vi "PH_AxisGUI_6P.PC_Information.vi"(0 "i ref in":refnum<vi>, 1 "quality":i32, 2 "Service Name":string, 3 "Axis Information":T2, 4 "no link":bool, 5 "error in":errorcluster) -> (14 "i ref out":refnum<vi>, 15 "Axis Selector":T1, 16 "Scaled Position":dbl, 19 "error out":errorcluster)   [LabVIEW 2014]
uses:
  PH_AxisGUI_6P.lvlib
  PH_Common/PH_Motion/PH_Motion.Axis State.ctl
  PH_AxisGUI_6P.AxisSelector.ctl
  PH_Common/PH_Motion/PH_Motion.Axis Activity.ctl
  PH_Common/PH_Motion/PH_Motion.Axis Information.ctl
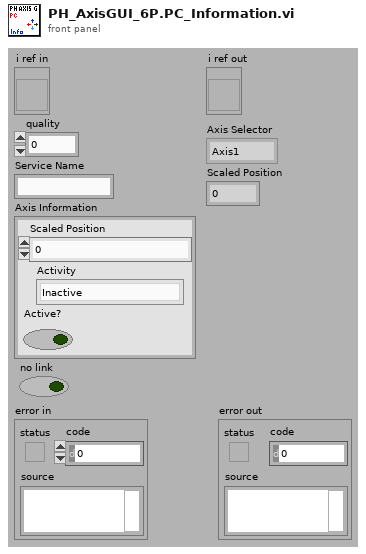
[diagram p1: front panel]
types:
  T1 = typedef "PH_AxisGUI_6P.lvlib/PH_AxisGUI_6P.AxisSelector.ctl" = enum16{"Axis1", "Axis2", "None"}
  T2 = typedef "PH_Motion.Axis Information.ctl" = cluster{"Scaled Position":dbl, "Activity":T3, "Active?":bool}
  T3 = typedef "PH_Motion.Axis Activity.ctl" = enum16{"Inactive", "Ramp", "PI-Controller", "Rotation", "Reference Switch Search", "Reference SwitchSearch", "Mechanical Reference"}
  T4 = typedef "PH_Motion.Axis State.ctl" = enum16{"NoLink", "Inactive", "Active", "Error", "NoInfo"}
  T5 = typedef "PH_AxisGUI_6P.lvlib/PH_AxisGUI_6P.i attribute.ctl" = cluster{"GUI Refs":cluster{"AxisSelection":refnum<vi>, "Tab Control":refnum<vi>}}
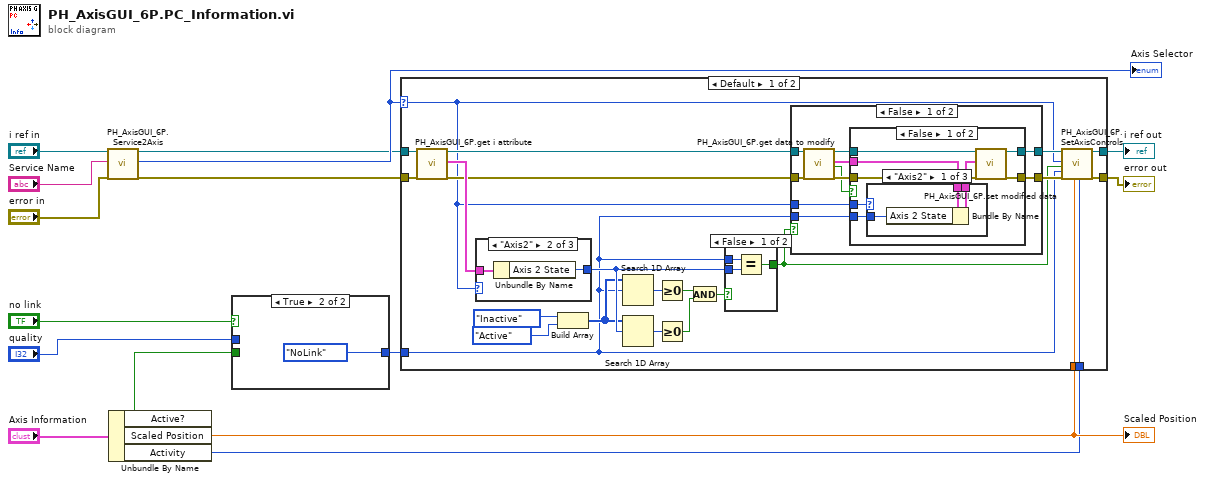
[diagram p0: block diagram]
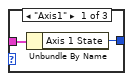
[diagram p2: hidden frame]
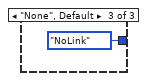
[diagram p3: hidden frame]
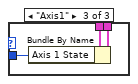
[diagram p5: hidden frame]
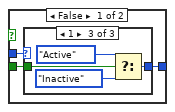
[diagram p10: hidden frame]
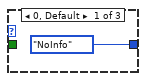
[diagram p11: hidden frame]
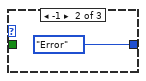
[diagram p12: hidden frame]
diagram:
  n1 = call "PH_AxisGUI_6P.Service2Axis.vi"("i ref in"="i ref in", "service name"="Service Name", "error in"="error in") -> ("i ref out"=w6:refnum<vi>, "Axis Selector"=w7:T1, "error out"=w5:errorcluster)  [unwired: 14 in]
  "Axis Selector" <- w7
  n2 = Unbundle By Name("Axis Information") -> ("Active?"=w10:bool, "Scaled Position"=w4:dbl, "Activity"=w3:T3)
  "Scaled Position" <- w4
  n3 = case "NO LINK?" shown="True" "no link" {
    tunnel: "quality" -> [w17 _]
    tunnel: [w18 PH_Motion.Axis_State."NoLink" ("AxisState")] -> w8
    tunnel: w10 -> [w16 _]
    frame False {
      n4 = case shown="1" w17 {
        tunnel: [PH_Motion.Axis_State."NoInfo" ("AxisState") PH_Motion.Axis_State."Error" ("AxisState") w24] -> w18
        tunnel: w16 -> [_ _ w21]
        frame 0, Default {
        }
        frame -1 {
        }
        frame 1 {
          n5 = Select(t=PH_Motion.Axis_State."Active" ("AxisState"), s=w21, f=PH_Motion.Axis_State."Inactive" ("AxisState")) -> (s? t:f=w24:T4)
        }
      }
    }
    frame True {
    }
  }
  n6 = case shown="Default" w7 {
    selector: w7 -> [w30 _]
    tunnel: w8 -> [w29 _]
    tunnel: w6 -> [w38 w88]
    tunnel: w5 -> [w36 w87]
    tunnel: [w34 w88] -> w1
    tunnel: [w32 w87] -> w2
    tunnel: w4 -> [w27 _]
    tunnel: w3 -> [w26 _]
    frame Default {
      n7 = call "PH_AxisGUI_6P.get i attribute.vi"("i ref in"=w38, "error in (no error)"=w36) -> ("i ref out"=w37:refnum<vi>, "i attribute"=w39:T5, "error out"=w35:errorcluster)  [unwired: 15 in]
      n8 = case shown="\"Axis2\"" w30 {
        tunnel: w39 -> [w50 w52 _]
        tunnel: [w49 w51 PH_Motion.Axis_State."NoLink" ("State")] -> w48
        frame "Axis1" {
          n9 = Unbundle By Name(w50) -> ("Axis 1 State"=w49:T4)
        }
        frame "Axis2" {
          n10 = Unbundle By Name(w52) -> ("Axis 2 State"=w51:T4)
        }
        frame "None", Default {
        }
      }
      n11 = Build Array(PH_Motion.Axis_State."Inactive" ("Axis1.State"), PH_Motion.Axis_State."Active" ("Axis1.State")) -> (w40:T4[])
      n12 = Search 1D Array(1D array=w40, element=w29) -> (index of element=w47:i32)  [unwired: 1 in]
      n13 = Search 1D Array(1D array=w40, element=w48) -> (index of element=w46:i32)  [unwired: 1 in]
      n14 = Greater Or Equal To 0?(x=w47) -> (x >= 0?=w45:bool)
      n15 = Greater Or Equal To 0?(x=w46) -> (x >= 0?=w44:bool)
      n16 = And(x=w45, y=w44) -> (x .and. y?=w43:bool)
      n17 = case shown="False" w43 {
        selector: w43 -> [_ w86]
        tunnel: [w85 w86] -> w28
        tunnel: w48 -> [w84 _]
        tunnel: w29 -> [w83 _]
        frame False {
          n18 = Equal?(x=w83, y=w84) -> (x = y?=w85:bool)
        }
        frame True {
        }
      }
      n19 = case shown="False" w28 {
        tunnel: w37 -> [w63 w82]
        tunnel: w35 -> [w61 w81]
        tunnel: [w59 w82] -> w33
        tunnel: [w58 w81] -> w31
        tunnel: w29 -> [w55 _]
        tunnel: w30 -> [w54 _]
        frame False {
          n20 = call "PH_AxisGUI_6P.get data to modify.vi"("i ref in"=w63, "error in (no error)"=w61) -> ("i ref out"=w62:refnum<vi>, "i attribute"=w56:T5, "timed out"=w57:bool, "error out"=w60:errorcluster)  [unwired: 14 in]
          n21 = case shown="False" w57 {
            tunnel: w62 -> [w71 w80]
            tunnel: w60 -> [w70 w79]
            tunnel: [w69 w80] -> w59
            tunnel: [w68 w79] -> w58
            tunnel: w56 -> [w67 _]
            tunnel: w55 -> [w65 _]
            tunnel: w54 -> [w64 _]
            frame False {
              n22 = case shown="\"Axis2\"" w64 {
                tunnel: w67 -> [w74 w75 w78]
                tunnel: [w73 w75 w77] -> w66
                tunnel: w65 -> [w72 _ w76]
                frame "Axis2" {
                  n23 = Bundle By Name(cluster=w74, "Axis 2 State"=w72) -> (w73:T5)
                }
                frame "None", Default {
                }
                frame "Axis1" {
                  n24 = Bundle By Name(cluster=w78, "Axis 1 State"=w76) -> (w77:T5)
                }
              }
              n25 = call "PH_AxisGUI_6P.set modified data.vi"("i ref in"=w71, "i attribute"=w66, "error in (no error)"=w70) -> ("i ref out"=w69:refnum<vi>, "error out"=w68:errorcluster)  [unwired: 15 in]
            }
            frame True {
            }
          }
        }
        frame True {
        }
      }
      n26 = call "PH_AxisGUI_6P.SetAxisControls.vi"("i ref in"=w33, "Axis Selector"=w30, "NoStateChanged"=w28, "State"=w29, "error in"=w31, "scaled Position"=w27, "Activity"=w26) -> ("i ref out"=w34:refnum<vi>, "error out"=w32:errorcluster)  [unwired: 11 in]
    }
    frame "None" {
    }
  }
  "error out" <- w2
  "i ref out" <- w1
